vi "Set_Alarm_Config.vi"(8 "error in (no error)":errorcluster, 11 "Alarm_Data In":T1) -> (0 "error out":errorcluster, 3 "Alarm_Data Out":T1)   [LabVIEW 2019, in "Alarm_Manager.lvlib"]
uses:
  Alarm_Manager.lvlib
  Alarm_Data.ctl
  Message_Handler/typedef/Alarm_Panel.ctl
  Channel_Temperature_Threshold.ctl
  Open_Circuit.ctl
  <vilib>/Utility/config.llb/Write Key (U32).vi
  <vilib>/Utility/config.llb/Write Key (I32).vi
  <vilib>/Utility/config.llb/NI_LVConfig.lvlib
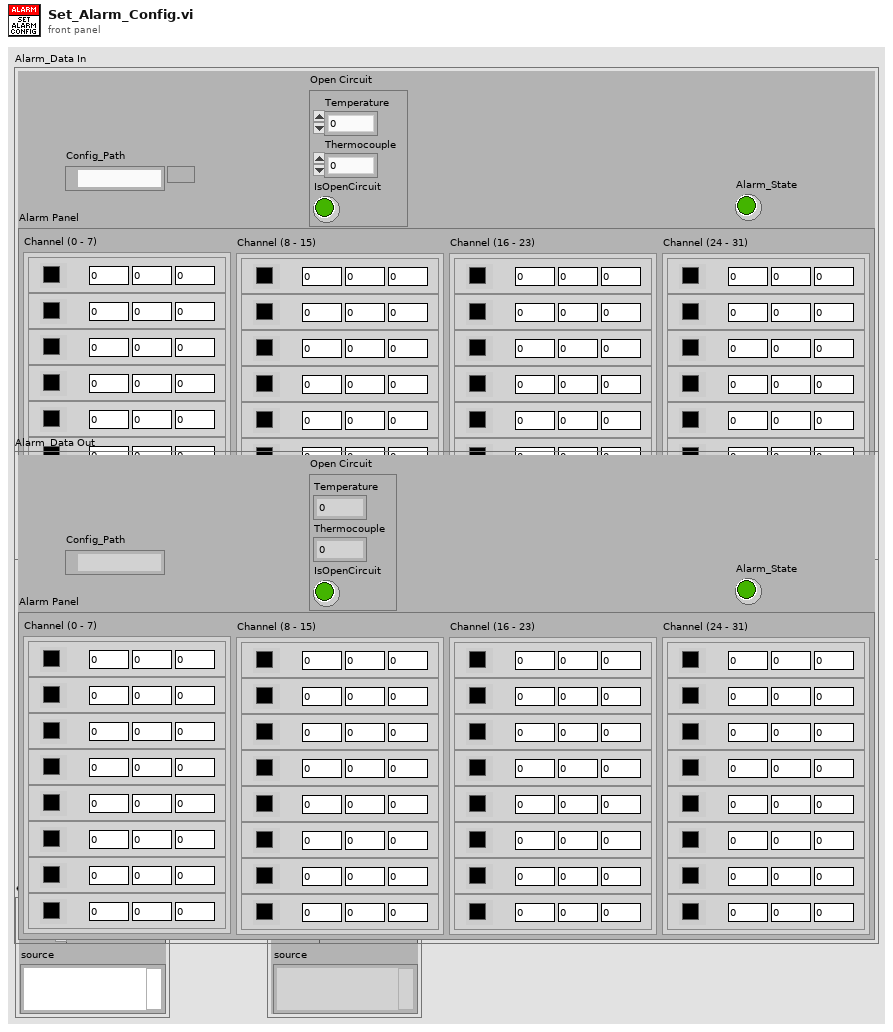
[diagram p1: front panel]
types:
  T1 = typedef "Alarm_Data.ctl" = cluster{"Alarm Panel":T2, "Alarm_State":bool, "Config_Path":path, "Open Circuit":T4}
  T2 = typedef "Alarm_Panel.ctl" = cluster{"Channel (0 - 7)":cluster{"Channel Temperature Thresholds":T3, "Channel Temperature Thresholds 2":T3, "Channel Temperature Thresholds 3":T3, "Channel Temperature Thresholds 4":T3, "Channel Temperature Thresholds 5":T3, "Channel Temperature Thresholds 6":T3, "Channel Temperature Thresholds 7":T3, "Channel Temperature Thresholds 8":T3}, "Channel (8 - 15)":cluster{"Channel Temperature Thresholds":T3, "Channel Temperature Thresholds 2":T3, "Channel Temperature Thresholds 3":T3, "Channel Temperature Thresholds 4":T3, "Channel Temperature Thresholds 5":T3, "Channel Temperature Thresholds 6":T3, "Channel Temperature Thresholds 7":T3, "Channel Temperature Thresholds 8":T3}, "Channel (16 - 23)":cluster{"Channel Temperature Thresholds":T3, "Channel Temperature Thresholds 2":T3, "Channel Temperature Thresholds 3":T3, "Channel Temperature Thresholds 4":T3, "Channel Temperature Thresholds 5":T3, "Channel Temperature Thresholds 6":T3, "Channel Temperature Thresholds 7":T3, "Channel Temperature Thresholds 8":T3}, "Channel (24 - 31)":cluster{"Channel Temperature Thresholds":T3, "Channel Temperature Thresholds 2":T3, "Channel Temperature Thresholds 3":T3, "Channel Temperature Thresholds 4":T3, "Channel Temperature Thresholds 5":T3, "Channel Temperature Thresholds 6":T3, "Channel Temperature Thresholds 7":T3, "Channel Temperature Thresholds 8":T3}}
  T3 = typedef "Channel_Temperature_Threshold.ctl" = cluster{"Min":i32, "Max":i32, "Alarm":i32, "Status":u32}
  T4 = typedef "Open_Circuit.ctl" = cluster{"Temperature":i32, "Thermocouple":i32, "IsOpenCircuit":bool}
  T5 = cluster{"Channel Temperature Thresholds":T3, "Channel Temperature Thresholds 2":T3, "Channel Temperature Thresholds 3":T3, "Channel Temperature Thresholds 4":T3, "Channel Temperature Thresholds 5":T3, "Channel Temperature Thresholds 6":T3, "Channel Temperature Thresholds 7":T3, "Channel Temperature Thresholds 8":T3}
  T6 = typedef "NI_LVConfig.lvlib/Config Data RefNum.ctl" = refnum<k1>
  T7 = cluster{"[0]":T3, "[1]":T3, "[2]":T3, "[3]":T3, "[4]":T3, "[5]":T3, "[6]":T3, "[7]":T3}
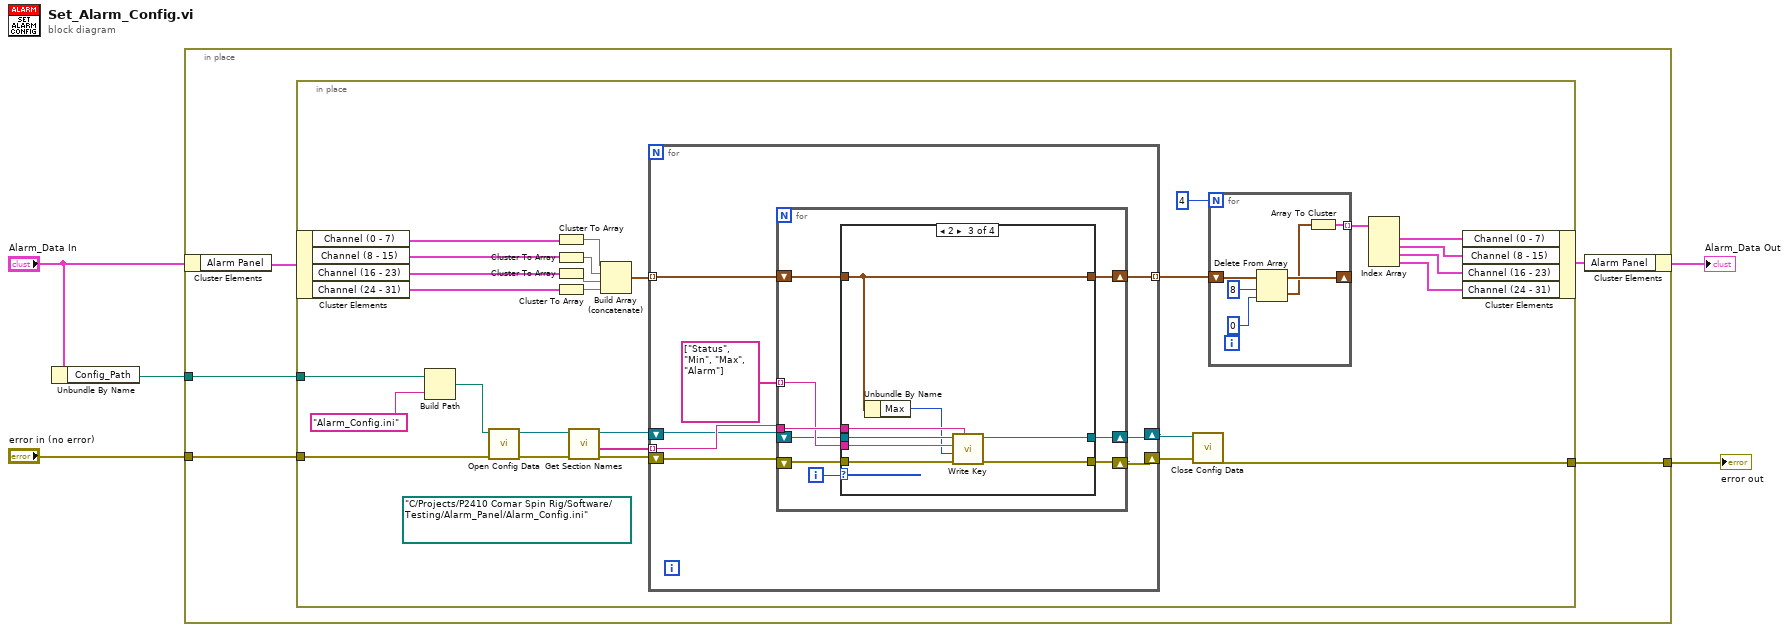
[diagram p0: block diagram]
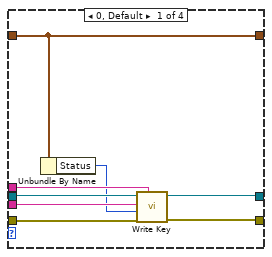
[diagram p2: hidden frame]
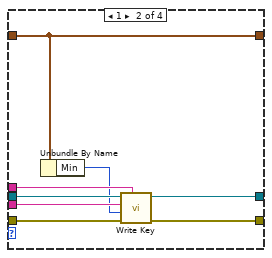
[diagram p3: hidden frame]
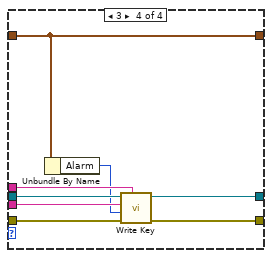
[diagram p4: hidden frame]
diagram:
  n1 = Unbundle By Name("Alarm_Data In") -> ("Config_Path"=w1:path)
  n2 = in-place {
    in-place-border: "error in (no error)" -> [w10]
    in-place-border: [w9] -> w4
    in-place-border: w1 -> [w6]
    n3 = in-place-cluster #1("Alarm_Data In") -> ("Alarm Panel"=w8:T2)
    n4 = in-place {
      in-place-border: w10 -> [w38]
      in-place-border: [w22] -> w9
      in-place-border: w6 -> [w13]
      (unwired) path "C:/Projects/P2410 Comar Spin Rig/Software/Testing/Alarm_Panel/Alarm_Config.ini" ("configuration file path")
      n5 = in-place-cluster #2(w8) -> ("Channel (0 - 7)"=w21:T5, "Channel (8 - 15)"=w20:T5, "Channel (16 - 23)"=w19:T5, "Channel (24 - 31)"=w18:T5)
      n6 = Build Path(base path=w13, name or relative path="Alarm_Config.ini") -> (appended path=w12:path)
      n7 = call <vilib>:"Open Config Data.vi"("error in (no error)"=w38, "configuration file path"=w12) -> ("error out"=w36:errorcluster, "refnum"=w37:T6)  [unwired: 7 in, 1 out]
      n8 = Cluster To Array(cluster=w21) -> (array=w29:T3[])
      n9 = Cluster To Array(cluster=w20) -> (array=w30:T3[])
      n10 = Cluster To Array(cluster=w19) -> (array=w31:T3[])
      n11 = Cluster To Array(cluster=w18) -> (array=w32:T3[])
      n12 = call <vilib>:"Get Section Names.vi"("error in (no error)"=w36, "refnum"=w37) -> ("error out"=w34:errorcluster, "section names"=w35:string[], "refnum out"=w33:T6)  [unwired: 7 in]
      n13 = Build Array (concatenate)(w29, w30, w31, w32) -> (w28:T3[])
      n14 = for {
        tunnel: w35 -> [w52] mode=indexing
        shift-right: [w50] -> w23
        shift-left: w34 -> [w51]
        shift-right: [w48] -> w24
        shift-left: w33 -> [w49]
        tunnel: w28 -> [w47] mode=indexing
        tunnel: [w46] -> w27 mode=indexing
        n15 = for {
          tunnel: w52 -> [w61]
          tunnel: string[] ["Status", "Min", "Max", "Alarm"] -> [w60] mode=indexing
          shift-right: [w58] -> w50
          shift-left: w51 -> [w59]
          shift-right: [w56] -> w48
          shift-left: w49 -> [w57]
          shift-right: [w53] -> w46
          shift-left: w47 -> [w54]
          i -> [w55]
          n16 = case shown="2" w55 {
            tunnel: w61 -> [w65 w77 w85 w93]
            tunnel: w60 -> [w64 w76 w84 w92]
            tunnel: w59 -> [w69 w75 w83 w91]
            tunnel: [w68 w74 w82 w90] -> w58
            tunnel: w57 -> [w66 w73 w81 w89]
            tunnel: [w67 w72 w80 w88] -> w56
            tunnel: w54 -> [w63 w71 w79 w87]
            tunnel: [w63 w71 w79 w87] -> w53
            frame 0, Default {
              n17 = Unbundle By Name(w63) -> ("Status"=w62:u32)
              n18 = call-poly <vilib>:"Write Key.vi"("section"=w65, "error in (no error)"=w69, "value"=w62, "key"=w64, "refnum"=w66) -> ("error out"=w68:errorcluster, "refnum out"=w67:T6)  [unwired: 4 in, 1 out]
            }
            frame 1 {
              n19 = Unbundle By Name(w71) -> ("Min"=w70:i32)
              n20 = call-poly <vilib>:"Write Key.vi"("section"=w77, "error in (no error)"=w75, "value"=w70, "key"=w76, "refnum"=w73) -> ("error out"=w74:errorcluster, "refnum out"=w72:T6)  [unwired: 4 in, 1 out]
            }
            frame 2 {
              n21 = Unbundle By Name(w79) -> ("Max"=w78:i32)
              n22 = call-poly <vilib>:"Write Key.vi"("section"=w85, "error in (no error)"=w83, "value"=w78, "key"=w84, "refnum"=w81) -> ("error out"=w82:errorcluster, "refnum out"=w80:T6)  [unwired: 4 in, 1 out]
            }
            frame 3 {
              n23 = Unbundle By Name(w87) -> ("Alarm"=w86:i32)
              n24 = call-poly <vilib>:"Write Key.vi"("section"=w93, "error in (no error)"=w91, "value"=w86, "key"=w92, "refnum"=w89) -> ("error out"=w90:errorcluster, "refnum out"=w88:T6)  [unwired: 4 in, 1 out]
            }
          }
        }
      }
      n25 = call <vilib>:"Close Config Data.vi"("error in (no error)"=w23, "refnum"=w24) -> ("error out"=w22:errorcluster)  [unwired: 8 in, 1 out]
      n26 = for {
        N: 4 -> [_]
        shift-right: [w42] -> _
        shift-left: w27 -> [w44]
        tunnel: [w39] -> w25 mode=indexing
        n27 = Delete From Array(array=w44, length=8, index=0) -> (deleted portion=w40:T3[], array with subset deleted=w42:T3[])
        n28 = Array To Cluster(array=w40) -> (cluster=w39:T7)
      }
      n29 = Index Array(array=w25) -> (element #1=w17:T7, element #2=w16:T7, element #3=w15:T7, element #4=w14:T7)  [unwired: 4 in]
      n30 = in-place-cluster #2("Channel (0 - 7)"=w17, "Channel (8 - 15)"=w16, "Channel (16 - 23)"=w15, "Channel (24 - 31)"=w14) -> (w7:T2)
    }
    n31 = in-place-cluster #1("Alarm Panel"=w7) -> (→"Alarm_Data Out":T1)
  }
  "error out" <- w4
